vi "Handle.vi"(8 "error in (no error)":errorcluster, 10 "Zero Timeout Message Handler in":refnum<class "Zero Timeout Message Handler.lvclass">, 11 "Message in":refnum<class "~Message.lvclass">) -> (0 "error out":errorcluster, 2 "Zero Timeout Message Handler out":refnum<class "Zero Timeout Message Handler.lvclass">)   [LabVIEW 2024, in "Zero Timeout Message Handler.lvlib" / "~Message.lvclass"]
uses:
  ~Message.lvclass
  Zero Timeout Message Handler/Zero Timeout Message Handler.lvclass
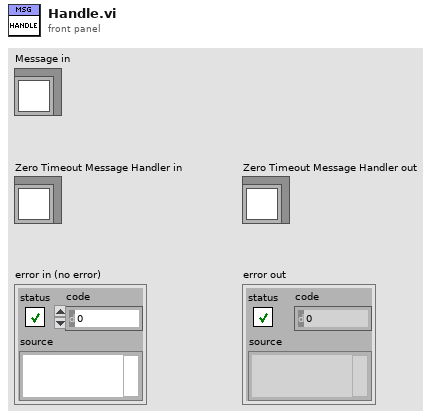
[diagram p1: front panel]
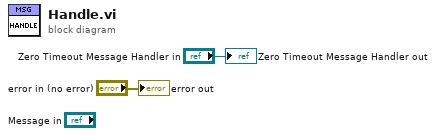
[diagram p0: block diagram]
diagram:
  "error out" <- "error in (no error)"
  "Zero Timeout Message Handler out" <- "Zero Timeout Message Handler in"
